vi "autoOff.vi"(8 "error in (no error)":errorcluster, 11 "Electrometer in":refnum<class "Electrometer.lvclass">) -> (0 "error out":errorcluster, 3 "Electrometer out":refnum<class "Electrometer.lvclass">)   [LabVIEW 2016, in "Electrometer.lvclass"]
uses:
  Electrometer.lvclass
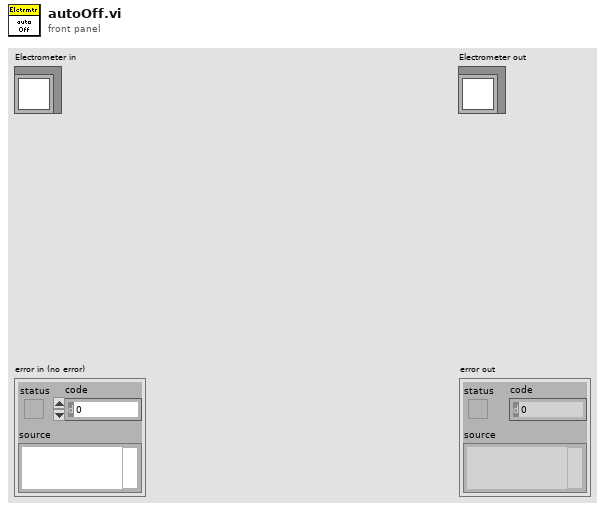
[diagram p1: front panel]
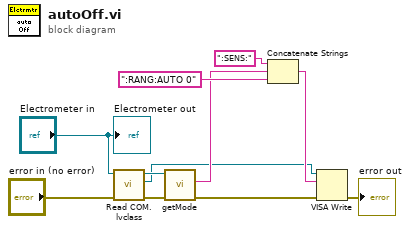
[diagram p0: block diagram]
diagram:
  n1 = call "Read COM.lvclass.vi"("error in (no error)"="error in (no error)", "Electrometer in"="Electrometer in") -> ("error out"=w4:errorcluster, "VISA"=w1:refnum<visa-resource-name>, "Electrometer out"=w5:refnum<class "Electrometer.lvclass">)  [unwired: 7 in]
  n2 = call "getMode.vi"("error in (no error)"=w4, "Electrometer in"=w5) -> ("error out"=w2:errorcluster, "Mode"=w3:string)  [unwired: 7 in, 1 out]
  n3 = Concatenate Strings(":SENS:", w3, ":RANG:AUTO 0" ("string")) -> (w8:string)
  n4 = VISA Write(VISA resource name=w1, write buffer=w8, error in (no error)=w2) -> (error out=→"error out":errorcluster)  [unwired: 2 out]
  "Electrometer out" <- "Electrometer in"
